vi "Lidar Down Sample.vi"(4 "Percentage of Lidar to be high":dbl=0.5, 5 "High Slice":dbl=2.0, 6 "Low Slice":dbl=10.0, 7 "Speed (m/s)":dbl=1.0, 8 "Speed Gain":dbl=1.0, 9 "Angle Array":dbl[](array[numeric]), 10 "Magnitude Array":dbl[](array[numeric])) -> (0 "Downsampled Angles":dbl[](array[numeric]), 3 "Downsamped Magnitudes":dbl[](array[numeric]))   [LabVIEW 2010]
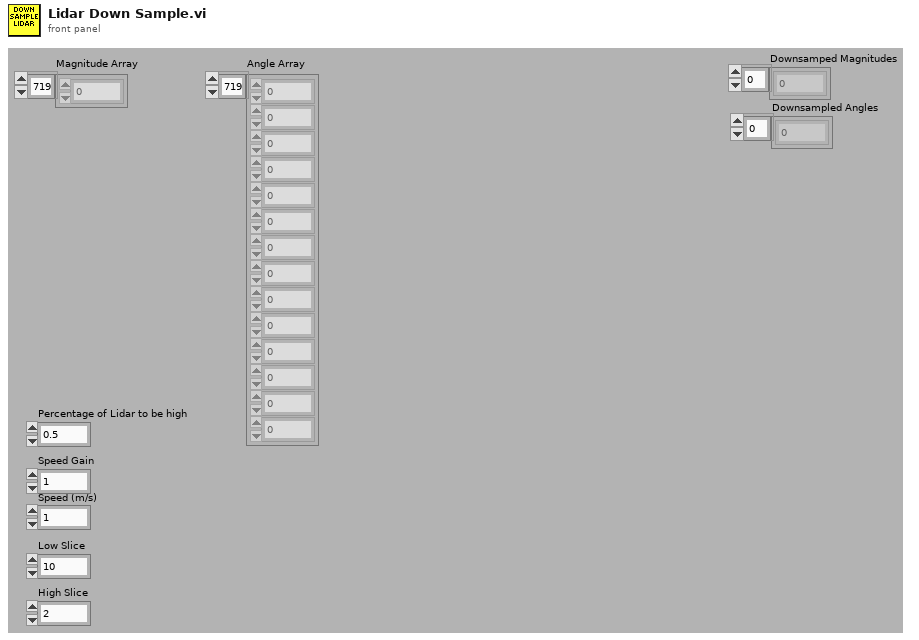
[diagram p1: front panel]
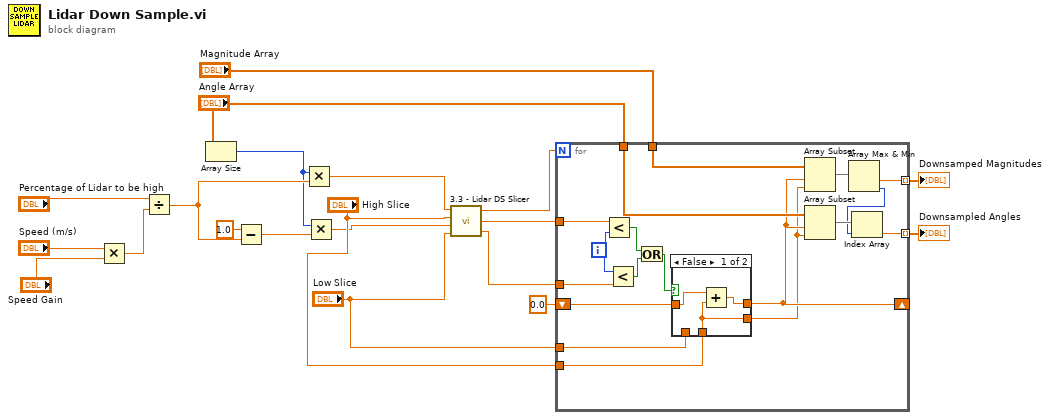
[diagram p0: block diagram]
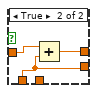
[diagram p2: hidden frame]
diagram:
  n1 = Multiply(x="Speed (m/s)", y="Speed Gain") -> (x*y=w18:dbl)
  n2 = Divide(x="Percentage of Lidar to be high", y=w18) -> (x/y=w15:dbl)
  n3 = Array Size(array="Angle Array") -> (size(s)=w14:i32)
  n4 = Subtract(x=1.0, y=w15) -> (x-y=w13:dbl)
  n5 = Multiply(x=w14, y=w15) -> (x*y=w8:dbl)
  n6 = Multiply(x=w14, y=w13) -> (x*y=w6:dbl)
  n7 = call "3.3 - Lidar DS Slicer.vi"("Low Slice"="Low Slice", "Numer of Cells to be low"=w6, "High Slice"="High Slice", "Numer of Cells to be high"=w8) -> ("Low lower bound"=w3:dbl, "Low upper bound"=w4:dbl, "Total iterations"=w9:dbl)
  n8 = for {
    N: w9 -> [_]
    tunnel: "Magnitude Array" -> [w38]
    tunnel: "Angle Array" -> [w37]
    tunnel: w3 -> [w30]
    tunnel: w4 -> [w29]
    tunnel: "Low Slice" -> [w34]
    tunnel: "High Slice" -> [w35]
    shift-right: [w33] -> _
    shift-left: 0.0 -> [w32]
    tunnel: [w23] -> w2 mode=indexing
    tunnel: [w21] -> w1 mode=indexing
    i -> [w28]
    n9 = Less?(x=w29, y=w28) -> (x < y?=w26:bool)
    n10 = Less?(x=w28, y=w30) -> (x < y?=w27:bool)
    n11 = Or(x=w26, y=w27) -> (x .or. y?=w36:bool)
    n12 = case shown="False" w36 {
      tunnel: w35 -> [w40 _]
      tunnel: w34 -> [_ w44]
      tunnel: [w40 w44] -> w31
      tunnel: [w41 w43] -> w33
      tunnel: w32 -> [w39 w42]
      frame False {
        n13 = Add(x=w39, y=w40) -> (x+y=w41:dbl)
      }
      frame True {
        n14 = Add(x=w42, y=w44) -> (x+y=w43:dbl)
      }
    }
    n15 = Array Subset(array=w38, index=w33, length=w31) -> (w25:dbl[])
    n16 = Array Subset(array=w37, index=w33, length=w31) -> (w24:dbl[])
    n17 = Array Max & Min(array=w25) -> (min value=w23:dbl, min index (indices)=w22:i32)  [unwired: 2 out]
    n18 = Index Array(array=w24, index=w22) -> (element=w21:dbl)
  }
  "Downsamped Magnitudes" <- w2
  "Downsampled Angles" <- w1
